vi "LVClass_HasoSlopes Apply Double Path.vi"(0 "HasoSlopes in":refnum<class "HasoSlopes.lvclass">, 7 "doublePath":T1, 11 "error in (no error)":errorcluster) -> (4 "HasoSlopes out":refnum<class "HasoSlopes.lvclass">, 15 "error out":errorcluster)   [LabVIEW 2020, in "HasoSlopes.lvclass"]
uses:
  HasoSlopes.lvclass
  SlopesPostProcessorList - Double passage.ctl
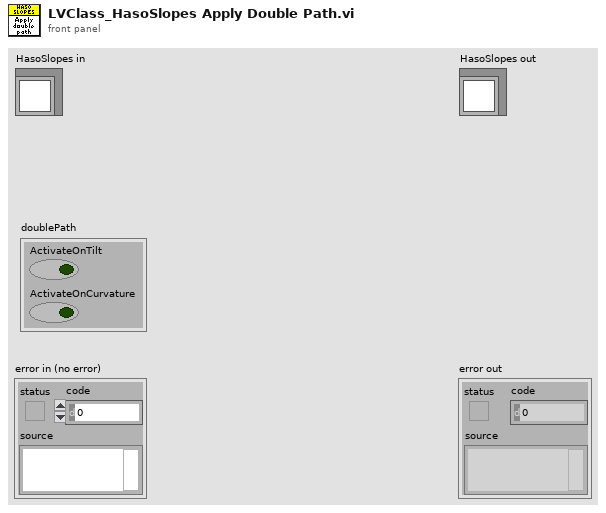
[diagram p1: front panel]
types:
  T1 = typedef "SlopesPostProcessorList - Double passage.ctl" = cluster{"ActivateOnTilt":bool, "ActivateOnCurvature":bool}
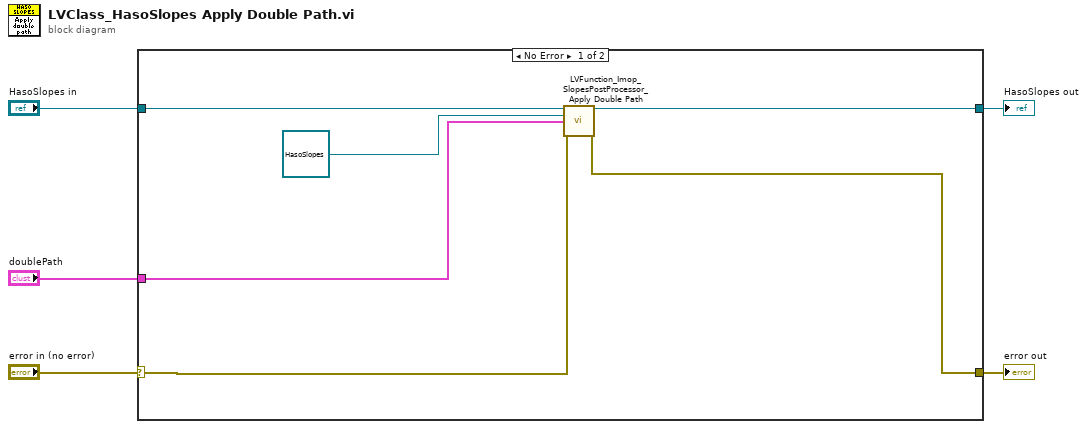
[diagram p0: block diagram]
diagram:
  n1 = case shown="No Error" "error in (no error)" {
    selector: "error in (no error)" -> [w9 w13]
    tunnel: [w8 w13] -> w4
    tunnel: [w10 w12] -> w2
    tunnel: "HasoSlopes in" -> [w11 w12]
    tunnel: "doublePath" -> [w7 _]
    frame No Error {
      n2 = call "LVFunction_Imop_SlopesPostProcessor_Apply Double Path.vi"("HasoSlopes in"=w11, "HasoSlopes OUT"=refnum<class "HasoSlopes.lvclass"> refnum, "doublePath"=w7, "error in (no error)"=w9) -> ("HasoSlopes out"=w10:refnum<class "HasoSlopes.lvclass">, "error out"=w8:errorcluster)  [unwired: 9 in, 1 out]
    }
    frame Error {
    }
  }
  "error out" <- w4
  "HasoSlopes out" <- w2
